vi "ELVIS III v1.0 RPC Undo Reserve Resouce.vi"(8 "error in (no error)":errorcluster, 10 "Channel Names":string[](array[string]), 11 "Session":u32) -> (0 "error out":errorcluster)   [LabVIEW 2021]
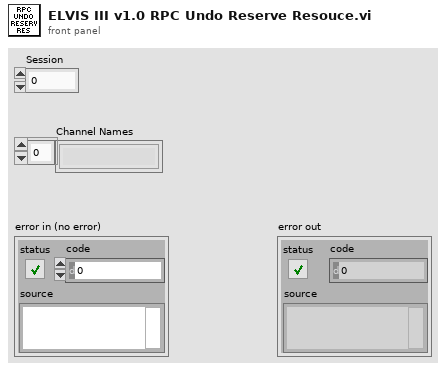
[diagram p1: front panel]
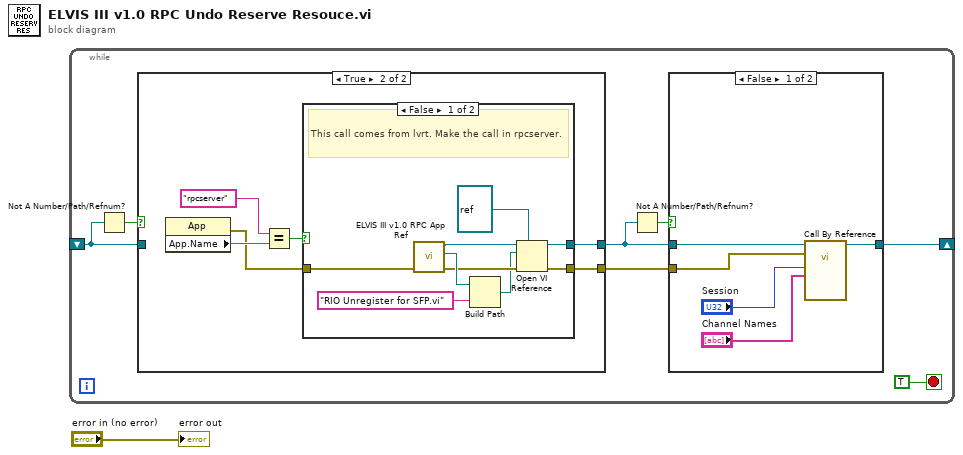
[diagram p0: block diagram]
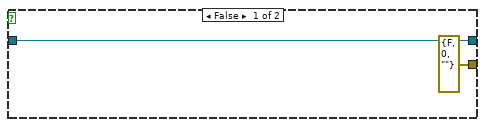
[diagram p2: hidden frame]
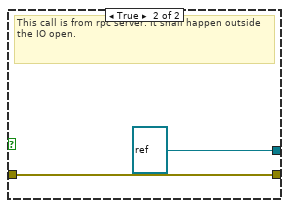
[diagram p3: hidden frame]
diagram:
  n1 = while {
    shift-right: [w5] -> _
    shift-left: _ -> [w3]
    stop <- TRUE stop-if-true
    n2 = Not A Number/Path/Refnum?(number/path/refnum=w3) -> (NaN/Path/Refnum?=w4:bool)
    n3 = case shown="True" w4 {
      tunnel: [w10 w13] -> w7
      tunnel: w3 -> [w10 _]
      tunnel: [errorcluster {"status"=FALSE, "code"=0, "source"=""} ("error out") w11] -> w2
      frame False {
      }
      frame True {
        n4 = property class="App"() -> (error out=w12:errorcluster, "App.Name"=w16:string)  [unwired: 2 in, 1 out]
        n5 = Equal?(x="rpcserver" ("Application:Name"), y=w16) -> (x = y?=w15:bool)
        n6 = case shown="False" w15 {
          tunnel: [w23 refnum<vi> refnum ("type specifier VI Refnum (for type only)")] -> w13
          tunnel: w12 -> [w18 w26]
          tunnel: [w22 w26] -> w11
          frame False {
            # "This call comes from lvrt. Make the call in rpcserver."
            n7 = call <vilib>:"ELVIS III v1.0 RPC App Ref.vi"() -> ("Lib Path"=w21:path, "RPC Reference"=w19:refnum<vi>)  [unwired: 10 in]
            n8 = Build Path(base path=w21, name or relative path="RIO Unregister for SFP.vi") -> (appended path=w17:path)
            n9 = Open VI Reference(type specifier VI Refnum (for type only)=refnum<vi> refnum, application reference (local)=w19, vi path=w17, error in (no error)=w18) -> (vi reference=w23:refnum<vi>, error out=w22:errorcluster)  [unwired: 2 in]
          }
          frame True {
            # "This call is from rpc server. It shall happen outside the IO open."
          }
        }
      }
    }
    n10 = Not A Number/Path/Refnum?(number/path/refnum=w7) -> (NaN/Path/Refnum?=w8:bool)
    n11 = case shown="False" w8 {
      tunnel: w7 -> [w31 w32]
      tunnel: [w30 w32] -> w5
      tunnel: w2 -> [w29 _]
      frame False {
        n12 = call-by-ref "?"(reference=w31, error in=w29, "Channel Names"="Channel Names", "Session"="Session") -> (reference out=w30:refnum<vi>)  [unwired: 9 in, 2 out]
      }
      frame True {
        # "The call is not available. The target is installed by 19.0. Ignore for backward compatibility."
      }
    }
  }
  "error out" <- "error in (no error)"
